vi "set y axis.vi"(11 "Array":dbl[][](array[numeric])) -> (2 "y multi":dbl, 3 "y offset":dbl)   [LabVIEW 2024]
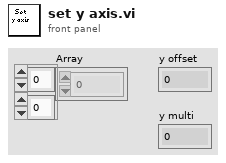
[diagram p1: front panel]
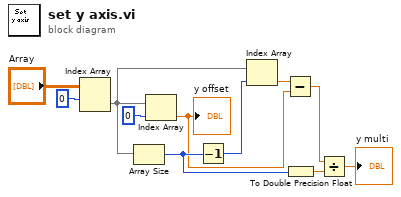
[diagram p0: block diagram]
diagram:
  n1 = Index Array(array="Array", index (row)=0) -> (element=w4:dbl[])  [unwired: 1 in]
  n2 = Array Size(array=w4) -> (size(s)=w9:i32)
  n3 = Index Array(array=w4, index=0) -> (element=w7:dbl)
  "y offset" <- w7
  n4 = Decrement(x=w9) -> (x-1=w5:i32)
  n5 = Index Array(array=w4, index=w5) -> (element=w6:dbl)
  n6 = Subtract(x=w6, y=w7) -> (x-y=w8:dbl)
  n7 = To Double Precision Float(number=w9) -> (double precision float=w10:dbl)
  n8 = Divide(x=w8, y=w10) -> (x/y=→"y multi":dbl)
